vi "AssignStatus_v2.vi"(4 "Time (s)":dbl, 5 "Rosco dt (s)":dbl, 6 "LoopCount":i32, 7 "Wind Estimator u(t=0) FS":dbl, 8 "error in (no error)":errorcluster, 9 "ROSCO Params In":T4, 10 "IO Signals In":T1, 11 "ArrayPairs In":T2={"iStatus"={"Index"=0, "Value"=0.0}, "TIME"={"Index"=1, "Value"=0.0}, "DT"={"Index"=2, "Value"=0.0}, "Blade1PitchPos_rad"={"Index"=3, "Value"=0.0}, "VS_MECHGENPWR"={"Index"=13, "Value"=0.0}, "VS_GENPWR"={"Index"=14, "Value"=0.0}, "GEN_SPEED"={"Index"=19, "Value"=0.0}, "ROTOR_SPEED"={"Index"=20, "Value"=0.0}, "GENTQMEAS"={"Index"=22, "Value"=0.0}, "Y_M"={"Index"=23, "Value"=0.0}, "HORWINDV"={"Index"=26, "Value"=0.0}, "ROOTMOOP1"={"Index"=29, "Value"=0.0}, "ROOTMOOP2"={"Index"=30, "Value"=0.0}, "Blade2PitchPos_rad"={"Index"=32, "Value"=0.0}, "Blade3PitchPos_rad"={"Index"=33, "Value"=0.0}, "ROOTMOOP3"={"Index"=31, "Value"=0.0}, "AVCMSG_SIZE"={"Index"=48, "Value"=0.0}, "INFILE_SIZE "={"Index"=49, "Value"=0.0}, "OUTFILE_SIZE "={"Index"=50, "Value"=0.0}, "FA_ACC"={"Index"=52, "Value"=0.0}, "NUM_BLADES"={"Index"=60, "Value"=0.0}, "BladePitchSetpoint_rad"={"Index"=44, "Value"=0.0}, "TorqueSetpoint_Nm"={"Index"=46, "Value"=0.0}, "OUT_AEROTQ"={"Index"=89, "Value"=0.0}, "Out.RotSpeed "={"Index"=92, "Value"=0.0}, "Out.DEBUG"={"Index"=93, "Value"=0.0}}) -> (0 "error out":errorcluster, 1 "ROSCO Params Out":T4, 2 "IO Signals Out":T1, 3 "ArrayPairs Out":T2={"iStatus"={"Index"=0, "Value"=0.0}, "TIME"={"Index"=1, "Value"=0.0}, "DT"={"Index"=2, "Value"=0.0}, "Blade1PitchPos_rad"={"Index"=3, "Value"=0.0}, "VS_MECHGENPWR"={"Index"=13, "Value"=0.0}, "VS_GENPWR"={"Index"=14, "Value"=0.0}, "GEN_SPEED"={"Index"=19, "Value"=0.0}, "ROTOR_SPEED"={"Index"=20, "Value"=0.0}, "GENTQMEAS"={"Index"=22, "Value"=0.0}, "Y_M"={"Index"=23, "Value"=0.0}, "HORWINDV"={"Index"=26, "Value"=0.0}, "ROOTMOOP1"={"Index"=29, "Value"=0.0}, "ROOTMOOP2"={"Index"=30, "Value"=0.0}, "Blade2PitchPos_rad"={"Index"=32, "Value"=0.0}, "Blade3PitchPos_rad"={"Index"=33, "Value"=0.0}, "ROOTMOOP3"={"Index"=31, "Value"=0.0}, "AVCMSG_SIZE"={"Index"=48, "Value"=0.0}, "INFILE_SIZE "={"Index"=49, "Value"=0.0}, "OUTFILE_SIZE "={"Index"=50, "Value"=0.0}, "FA_ACC"={"Index"=52, "Value"=0.0}, "NUM_BLADES"={"Index"=60, "Value"=0.0}, "BladePitchSetpoint_rad"={"Index"=44, "Value"=0.0}, "TorqueSetpoint_Nm"={"Index"=46, "Value"=0.0}, "OUT_AEROTQ"={"Index"=89, "Value"=0.0}, "Out.RotSpeed "={"Index"=92, "Value"=0.0}, "Out.DEBUG"={"Index"=93, "Value"=0.0}})   [LabVIEW 2018]
uses:
  Clusters/RoscoParams.ctl
  Clusters/ArrayPairs.ctl
  Clusters/SwapArrayCluster.ctl
  Clusters/IOSignals.ctl
  Clusters/SimulationConstants.ctl
  Clusters/ScalingEnum.ctl
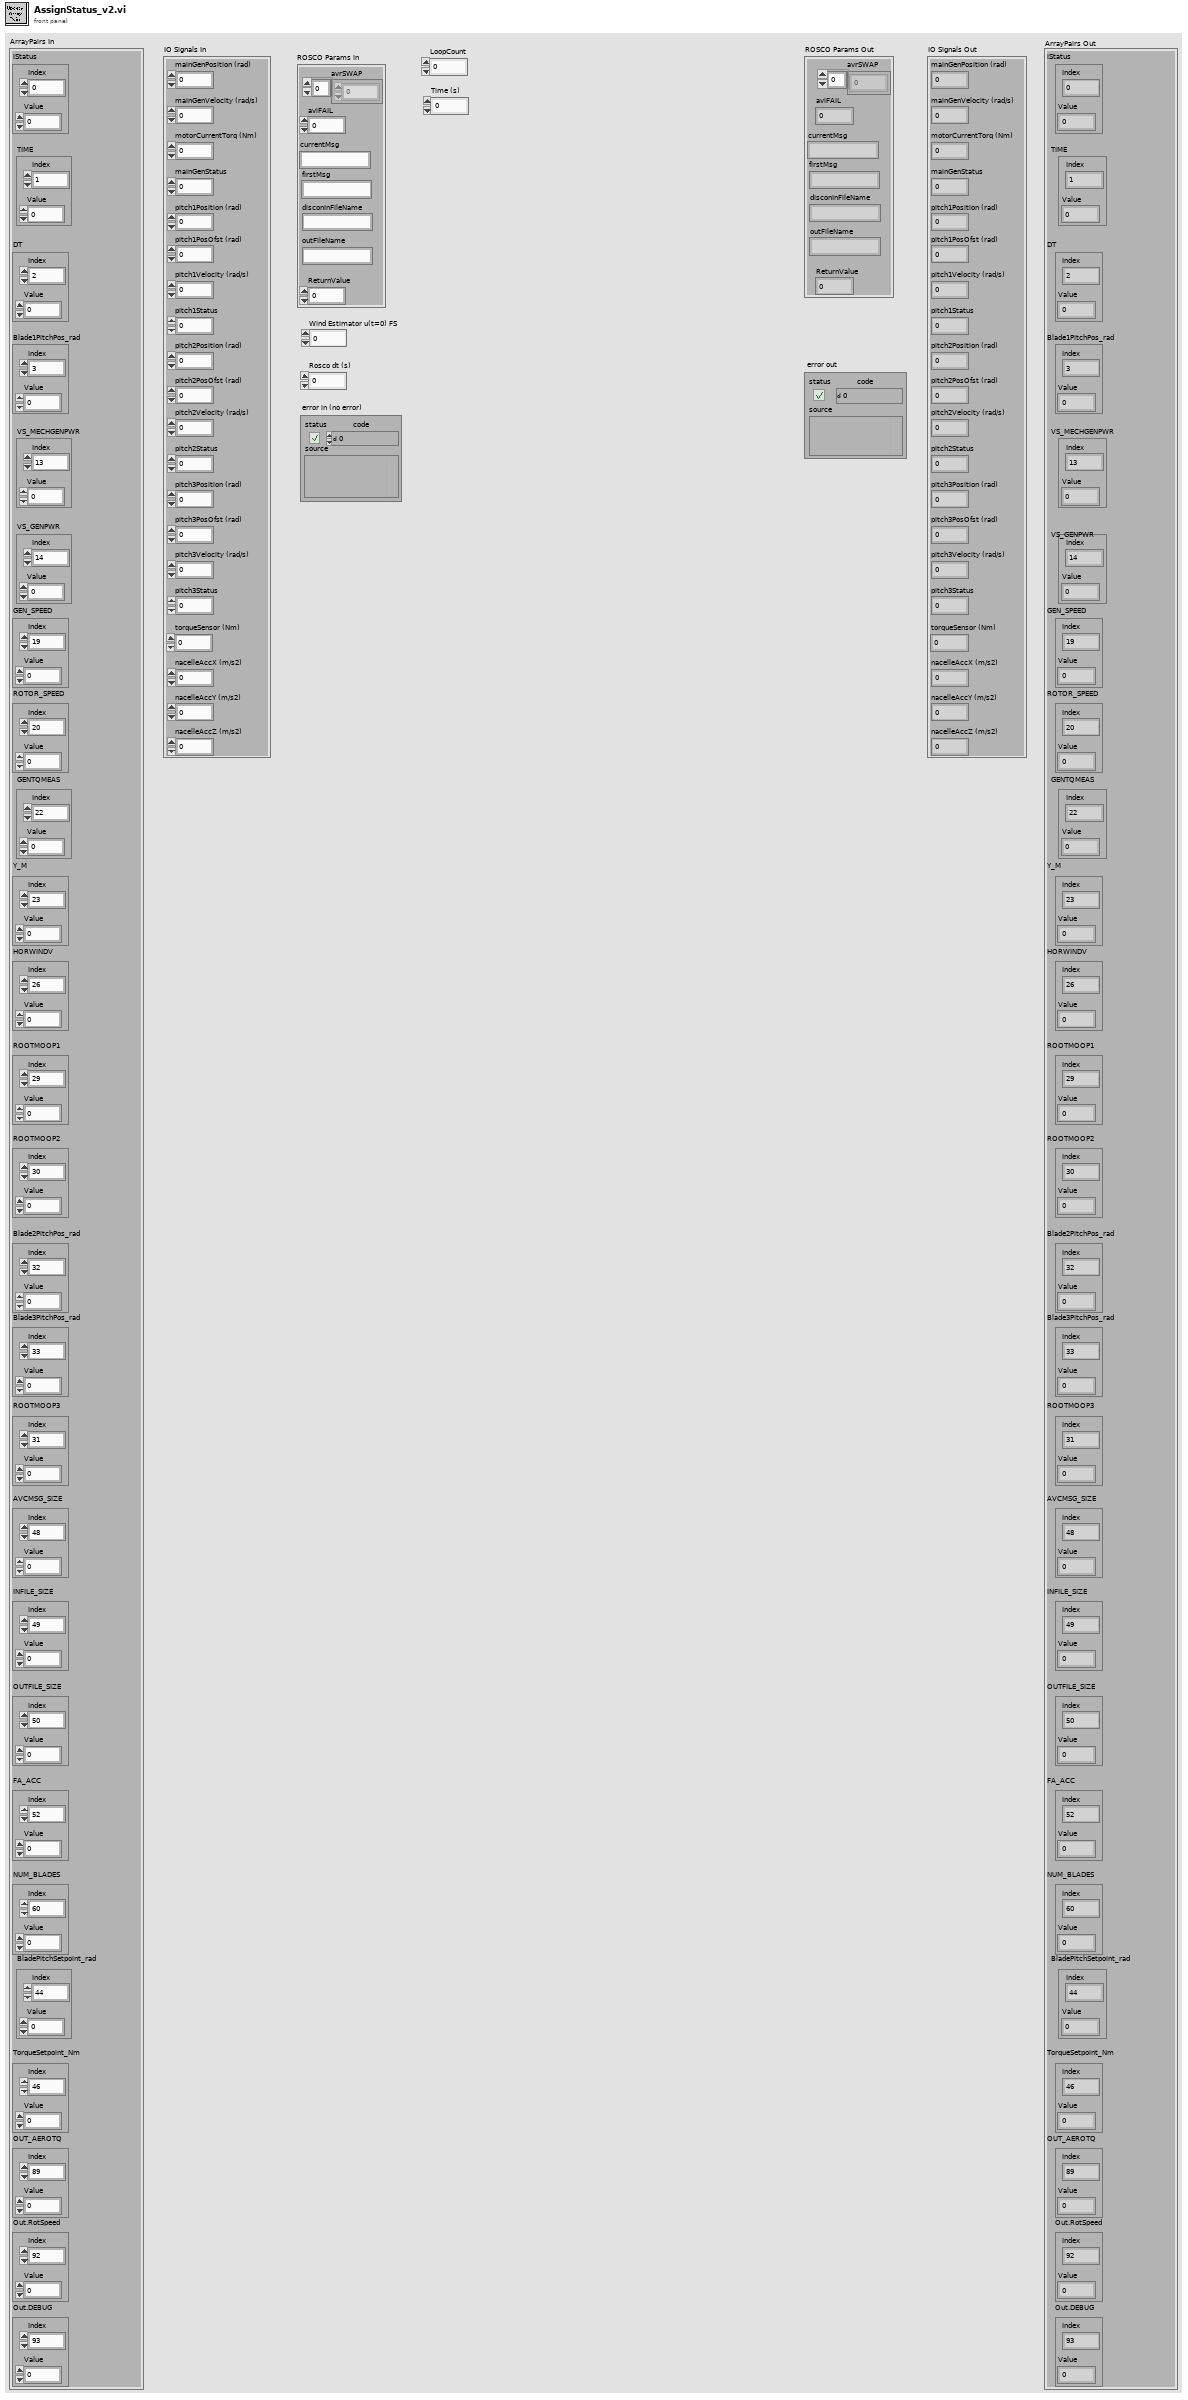
[diagram p1: front panel]
types:
  T1 = typedef "IOSignals.ctl" = cluster{"mainGenPosition (rad)":dbl, "motorCurrentTorq (Nm)":dbl, "mainGenVelocity (rad/s)":dbl, "mainGenStatus":u16, "pitch1Position (rad)":dbl, "pitch1Velocity (rad/s)":dbl, "pitch1Status":u16, "pitch2Position (rad)":dbl, "pitch2Velocity (rad/s)":dbl, "pitch2Status":u16, "pitch3Position (rad)":dbl, "pitch3Velocity (rad/s)":dbl, "pitch3Status":u16, "pitch1PosOfst (rad)":dbl, "pitch2PosOfst (rad)":dbl, "pitch3PosOfst (rad)":dbl, "torqueSensor (Nm)":dbl, "nacelleAccX (m/s2)":dbl, "nacelleAccY (m/s2)":dbl, "nacelleAccZ (m/s2)":dbl}
  T2 = typedef "ArrayPairs.ctl" = cluster{"iStatus":T3, "TIME":T3, "DT":T3, "Blade1PitchPos_rad":T3, "VS_MECHGENPWR":T3, "VS_GENPWR":T3, "GEN_SPEED":T3, "ROTOR_SPEED":T3, "GENTQMEAS":T3, "Y_M":T3, "HORWINDV":T3, "ROOTMOOP1":T3, "ROOTMOOP2":T3, "Blade2PitchPos_rad":T3, "Blade3PitchPos_rad":T3, "ROOTMOOP3":T3, "AVCMSG_SIZE":T3, "INFILE_SIZE ":T3, "OUTFILE_SIZE ":T3, "FA_ACC":T3, "NUM_BLADES":T3, "BladePitchSetpoint_rad":T3, "TorqueSetpoint_Nm":T3, "OUT_AEROTQ":T3, "Out.RotSpeed ":T3, "Out.DEBUG":T3}
  T3 = typedef "SwapArrayCluster.ctl" = cluster{"Index":i32, "Value":dbl}
  T4 = typedef "RoscoParams.ctl" = cluster{"avrSWAP":dbl[], "aviFAIL":i32, "currentMsg":string, "ReturnValue":i32, "disconInFileName":string, "outFileName":string, "firstMsg":string}
  T5 = typedef "ScalingEnum.ctl" = enum16{"Model scale -> Full scale", "Full scale -> Model scale"}
  T6 = typedef "SimulationConstants.ctl" = cluster{"Ngear":dbl, "GeneratorEff":dbl, "RotorRadius":sgl, "NumBlades":i32, "ScaleFactor":dbl, "RoscoInit min speed (rad/s)":dbl, "RoscoInit min torque (Nm) FS":dbl}
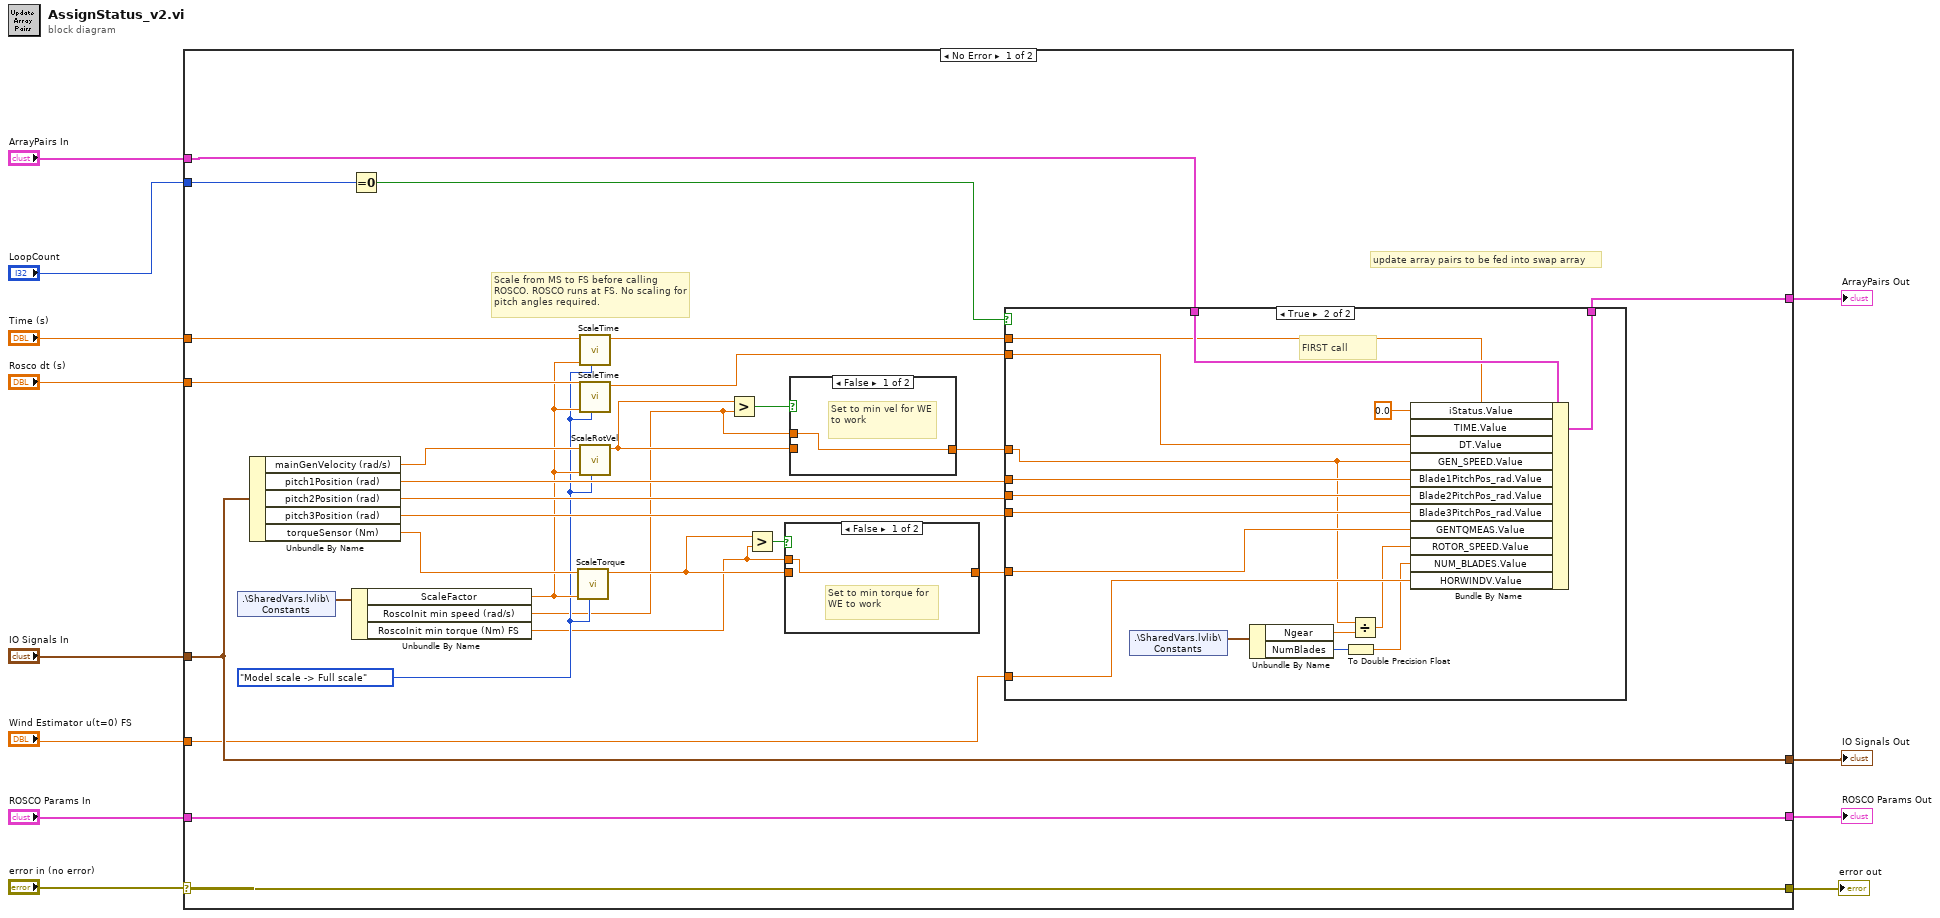
[diagram p0: block diagram]
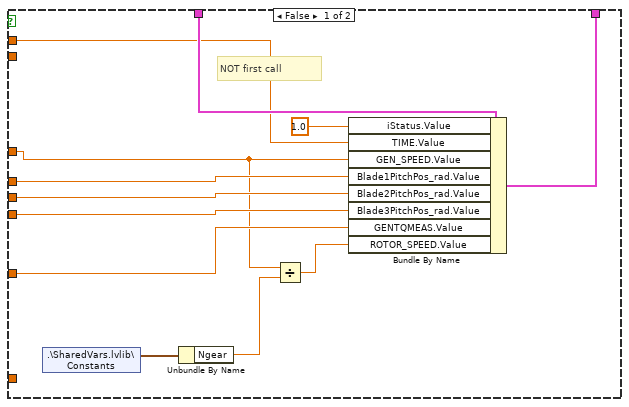
[diagram p4: hidden frame]
diagram:
  n1 = case shown="No Error" "error in (no error)" {
    selector: "error in (no error)" -> [w40 w76]
    tunnel: [w39 w75] -> w5
    tunnel: "LoopCount" -> [w38 _]
    tunnel: [w40 w76] -> w10
    tunnel: [w34 w74] -> w8
    tunnel: "ROSCO Params In" -> [w34 w74]
    tunnel: "ArrayPairs In" -> [w33 w75]
    tunnel: "Time (s)" -> [w29 _]
    tunnel: "IO Signals In" -> [w36 w73]
    tunnel: [w36 w73] -> w3
    tunnel: "Wind Estimator u(t=0) FS" -> [w35 _]
    tunnel: "Rosco dt (s)" -> [w27 _]
    frame No Error {
      w21 = ScalingEnum."Model scale -> Full scale" ("Scale Dir")
      # "Scale from MS to FS before calling ROSCO. ROSCO runs at FS. No scaling for pitch angles required."
      # "update array pairs to be fed into swap array"
      n2 = shared-variable ".\\SharedVars.lvlib\\Constants"() -> (w23:T6)  [unwired: 1 in, 1 out]
      n3 = Unbundle By Name(w36) -> ("mainGenVelocity (rad/s)"=w25:dbl, "pitch1Position (rad)"=w32:dbl, "pitch2Position (rad)"=w31:dbl, "pitch3Position (rad)"=w30:dbl, "torqueSensor (Nm)"=w24:dbl)
      n4 = Equal To 0?(x=w38) -> (x = 0?=w37:bool)
      n5 = Unbundle By Name(w23) -> ("ScaleFactor"=w22:dbl, "RoscoInit min speed (rad/s)"=w14:dbl, "RoscoInit min torque (Nm) FS"=w13:dbl)
      n6 = call "ScaleTorque.vi"("Scale Dir"=w21, "Scale factor"=w22, "Torque (In)"=w24) -> ("Torque (Out)"=w16:dbl)  [unwired: 8 in]
      n7 = call "ScaleTime.vi"("Scale Dir"=w21, "Scale factor"=w22, "Time (In)"=w29) -> ("Time OUT (Out)"=w28:dbl)  [unwired: 8 in]
      n8 = call "ScaleTime.vi"("Scale Dir"=w21, "Scale factor"=w22, "Time (In)"=w27) -> ("Time OUT (Out)"=w26:dbl)  [unwired: 8 in]
      n9 = call "ScaleRotVel.vi"("Scale Dir"=w21, "Scale factor"=w22, "Rotational Velocity (In)"=w25) -> ("Rotational Velocity (Out)"=w19:dbl)  [unwired: 8 in]
      n10 = Greater?(x=w19, y=w14) -> (0:w20:bool)
      n11 = Greater?(x=w16, y=w13) -> (0:w17:bool)
      n12 = case shown="False" w17 {
        tunnel: w16 -> [_ w42]
        tunnel: [w41 w42] -> w15
        tunnel: w13 -> [w41 _]
        frame False {
          # "Set to min torque for WE to work"
        }
        frame True {
          # "Pass through"
        }
      }
      n13 = case shown="False" w20 {
        tunnel: w19 -> [_ w44]
        tunnel: [w43 w44] -> w18
        tunnel: w14 -> [w43 _]
        frame False {
          # "Set to min vel for WE to work"
        }
        frame True {
          # "Pass through"
        }
      }
      n14 = case shown="True" w37 {
        tunnel: w33 -> [w56 w72]
        tunnel: [w55 w71] -> w39
        tunnel: w28 -> [w53 w69]
        tunnel: w35 -> [_ w67]
        tunnel: w32 -> [w50 w59]
        tunnel: w31 -> [w49 w60]
        tunnel: w30 -> [w48 w61]
        tunnel: w15 -> [w47 w62]
        tunnel: w26 -> [_ w58]
        tunnel: w18 -> [w45 w57]
        frame False {
          # "NOT first call"
          n15 = shared-variable ".\\SharedVars.lvlib\\Constants"() -> (w46:T6)  [unwired: 1 in, 1 out]
          n16 = Unbundle By Name(w46) -> ("Ngear"=w52:dbl)
          n17 = Divide(x=w45, y=w52) -> (x/y=w51:dbl)
          n18 = Bundle By Name(cluster=w56, "iStatus.Value"=1.0, "TIME.Value"=w53, "GEN_SPEED.Value"=w45, "Blade1PitchPos_rad.Value"=w50, "Blade2PitchPos_rad.Value"=w49, "Blade3PitchPos_rad.Value"=w48, "GENTQMEAS.Value"=w47, "ROTOR_SPEED.Value"=w51) -> (w55:T2)
        }
        frame True {
          # "FIRST call"
          n19 = shared-variable ".\\SharedVars.lvlib\\Constants"() -> (w65:T6)  [unwired: 1 in, 1 out]
          n20 = Unbundle By Name(w65) -> ("Ngear"=w68:dbl, "NumBlades"=w66:i32)
          n21 = To Double Precision Float(number=w66) -> (double precision float=w64:dbl)
          n22 = Divide(x=w57, y=w68) -> (x/y=w63:dbl)
          n23 = Bundle By Name(cluster=w72, "iStatus.Value"=0.0, "TIME.Value"=w69, "DT.Value"=w58, "GEN_SPEED.Value"=w57, "Blade1PitchPos_rad.Value"=w59, "Blade2PitchPos_rad.Value"=w60, "Blade3PitchPos_rad.Value"=w61, "GENTQMEAS.Value"=w62, "ROTOR_SPEED.Value"=w63, "NUM_BLADES.Value"=w64, "HORWINDV.Value"=w67) -> (w71:T2)
        }
      }
    }
    frame Error {
    }
  }
  "error out" <- w10
  "ROSCO Params Out" <- w8
  "ArrayPairs Out" <- w5
  "IO Signals Out" <- w3
